vi "Actor Setup.vi"(10 "Self Actor":refnum<class "Actor.lvclass">, 11 "Process in":refnum<class "ABD.lvclass">) -> (0 "error out":errorcluster, 3 "Process out":refnum<class "ABD.lvclass">)   [LabVIEW 2021, in "ABD.lvlib" / "ABD.lvclass"]
uses:
  ABD.lvclass
  LVCAM/LVCAM/Actor/Actor.lvclass
  ABD Panel/ABD Panel.lvclass
  C:/PPLs/LabVIEW-Composed-Actor-Model-LVCAM/LabVIEW-Composed-Actor-Model-LVCAM/Panel/Panel.lvclass
  ABD.lvclass/ABD.ctl
  Panel/Panel.lvclass
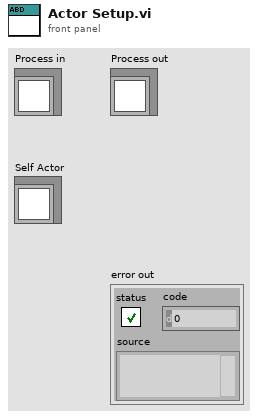
[diagram p1: front panel]
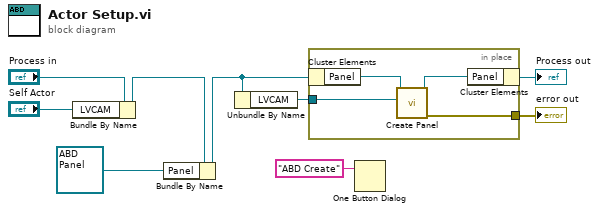
[diagram p0: block diagram]
diagram:
  n1 = Bundle By Name(cluster="Process in", "LVCAM"="Self Actor") -> (w4:refnum<class "ABD.lvclass">)
  n2 = Bundle By Name(cluster=w4, "Panel"=refnum<class "ABD Panel.lvclass"> refnum ("ABD Panel.lvclass")) -> (w2:refnum<class "ABD.lvclass">)
  n3 = Unbundle By Name(w2) -> ("LVCAM"=w3:refnum<class "Actor.lvclass">)
  n4 = in-place {
    in-place-border: [w11] -> w5
    in-place-border: w3 -> [w10]
    n5 = in-place-cluster #1(w2) -> ("Panel"=w13:refnum<class "Panel.lvclass">)
    n6 = call "Create Panel.vi"("LVCAM"=w10, "Panel in"=w13) -> ("error out"=w11:errorcluster, "Panel out"=w12:refnum<class "Panel.lvclass">)  [unwired: 8 in]
    n7 = in-place-cluster #1("Panel"=w12) -> (→"Process out":refnum<class "ABD.lvclass">)
  }
  "error out" <- w5
  n8 = One Button Dialog(message="ABD Create") -> ()  [unwired: 1 in, 1 out]
